vi "Get Project Members from Path - SM.vi"(6 "Shallow Scan":bool, 7 "AppRef":refnum<vi>, 8 "error in":errorcluster, 11 "Project Path":path) -> (0 "error out":errorcluster, 2 "Project Members":path[](array[path]))   [LabVIEW 2009, in "GraphicalTestRunner.lvlib"]
uses:
  GraphicalTestRunner.lvlib
  <userlib>/_OpenG.lib/array/array.llb/Remove Duplicates from 1D Array (Path)__ogtk.vi
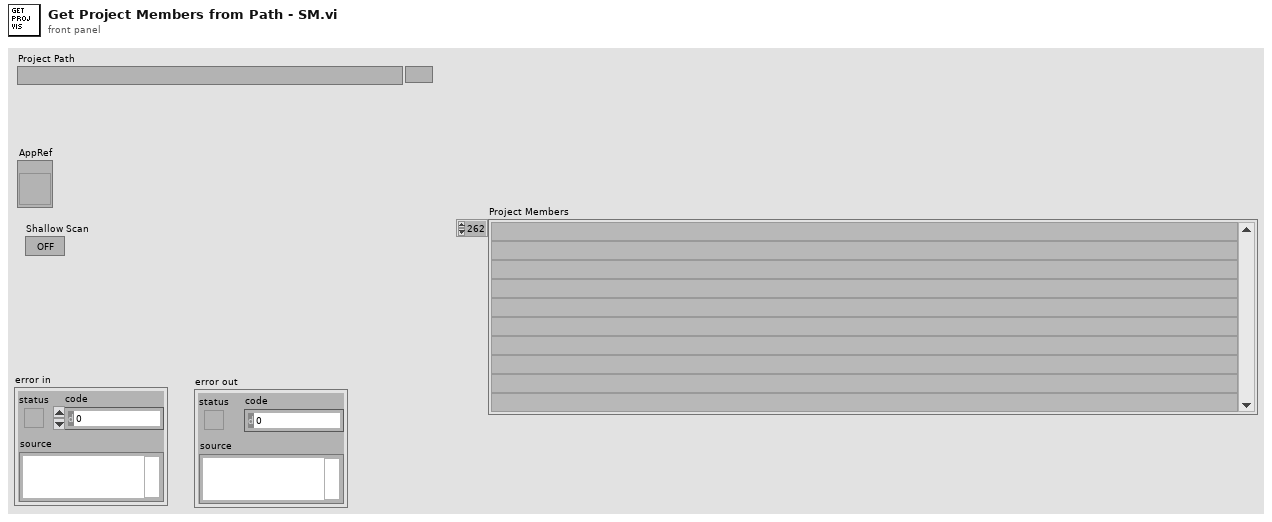
[diagram p1: front panel]
types:
  T1 = enum32{"Invalid", "Standard", "Closed", "Hidden", "Minimized", "Maximized"}
  T2 = enum32{"invalid app kind", "Development System", "Run Time System", "Student Edition", "Embedded LabVIEW", "Evaluation", "Custom"}
  T3 = cluster{"Current VI Reference":refnum<vi>, "AppRef":refnum<vi>, "Project":refnum<vi>, "My Computer":refnum<vi>, "Shallow Scan":bool, "Project Members":path[]}
  T4 = typedef "Liner Info - Cluster__jki_lib_application_control.ctl" = cluster{"path":path, "type":enum32{"Instrument", "Control", "CIN", "External subroutine", "Shared library", "Run-time menu", "Help file", "Palette menu"}, "iState":u32, "iStyle":u16, "wStyle":u16, "buttons":u16, "viflags":u32, "viflags2":u32, "links":u32[]}
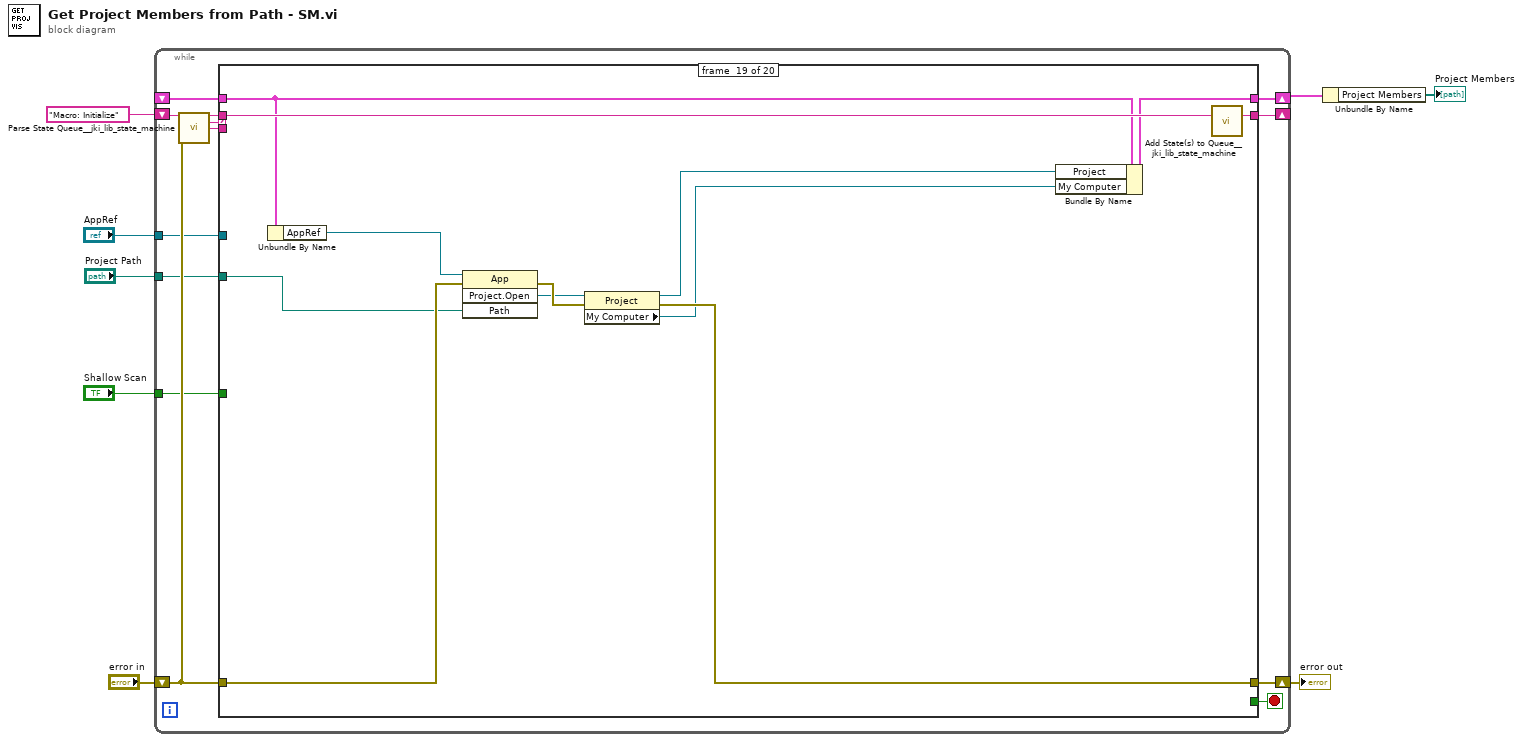
[diagram p0: block diagram]
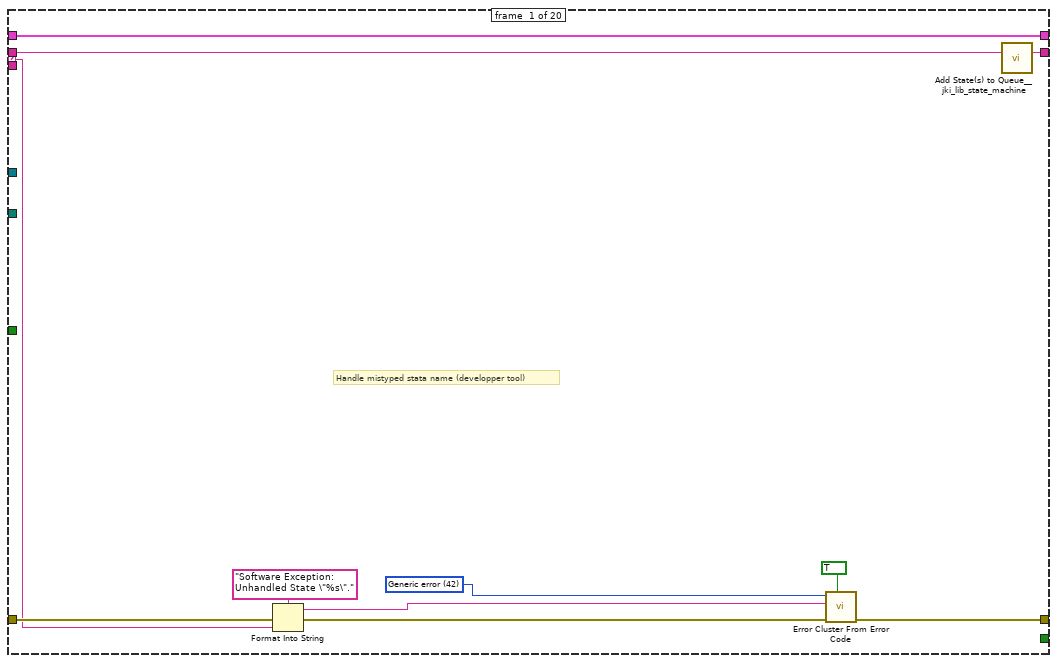
[diagram p2: hidden frame]
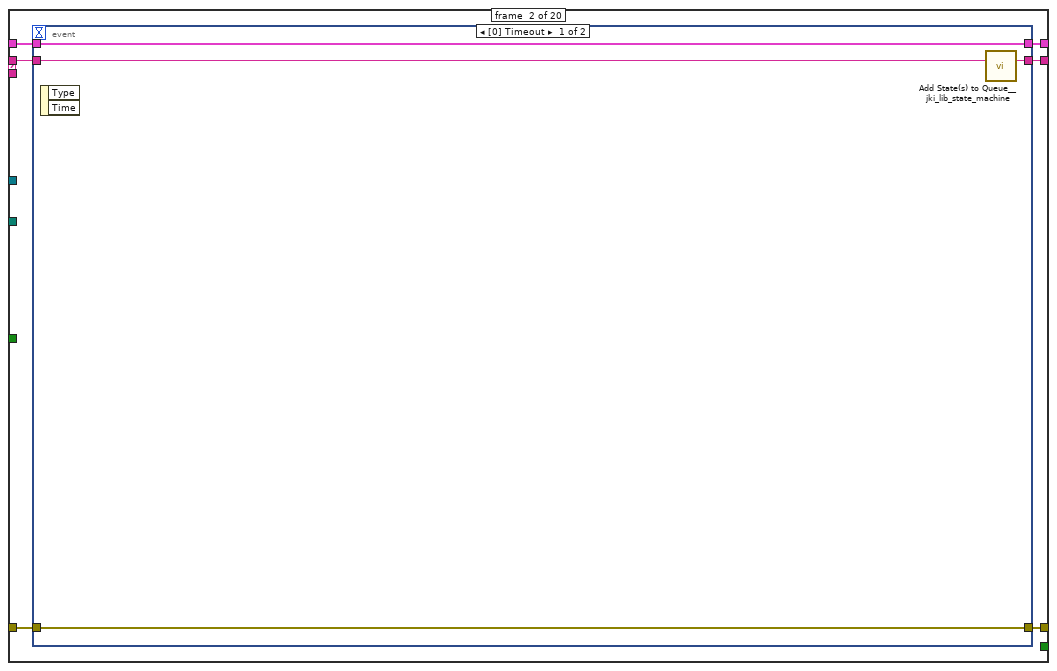
[diagram p3: hidden frame]
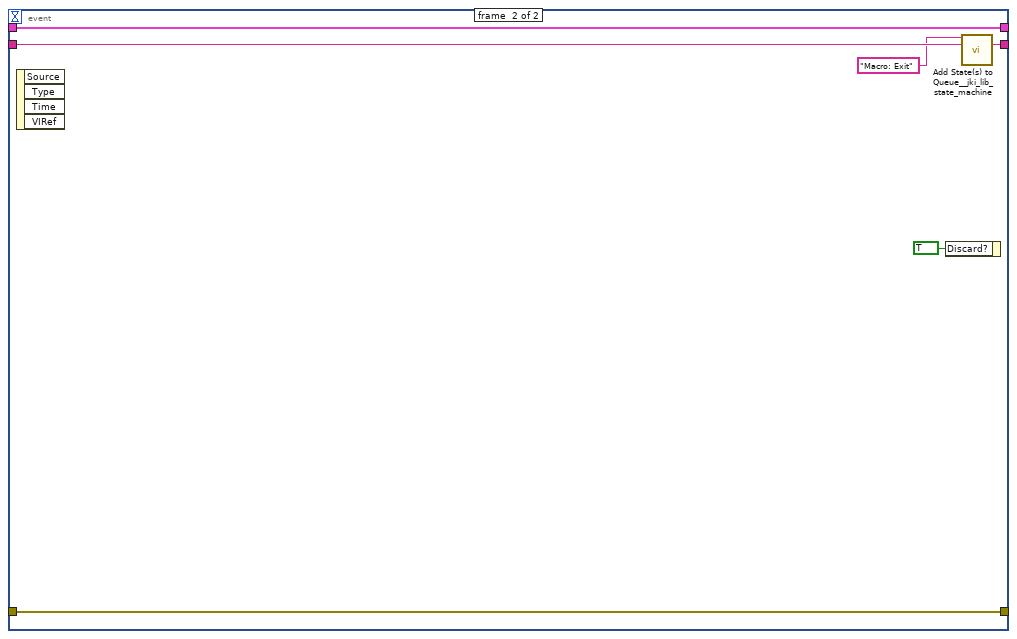
[diagram p4: hidden frame]
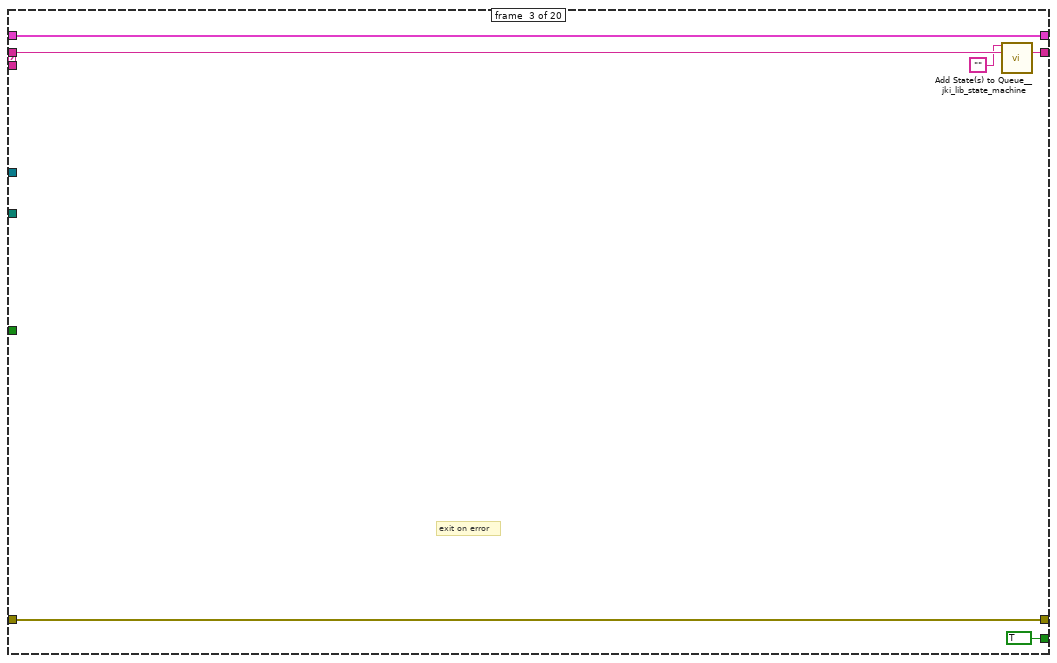
[diagram p5: hidden frame]
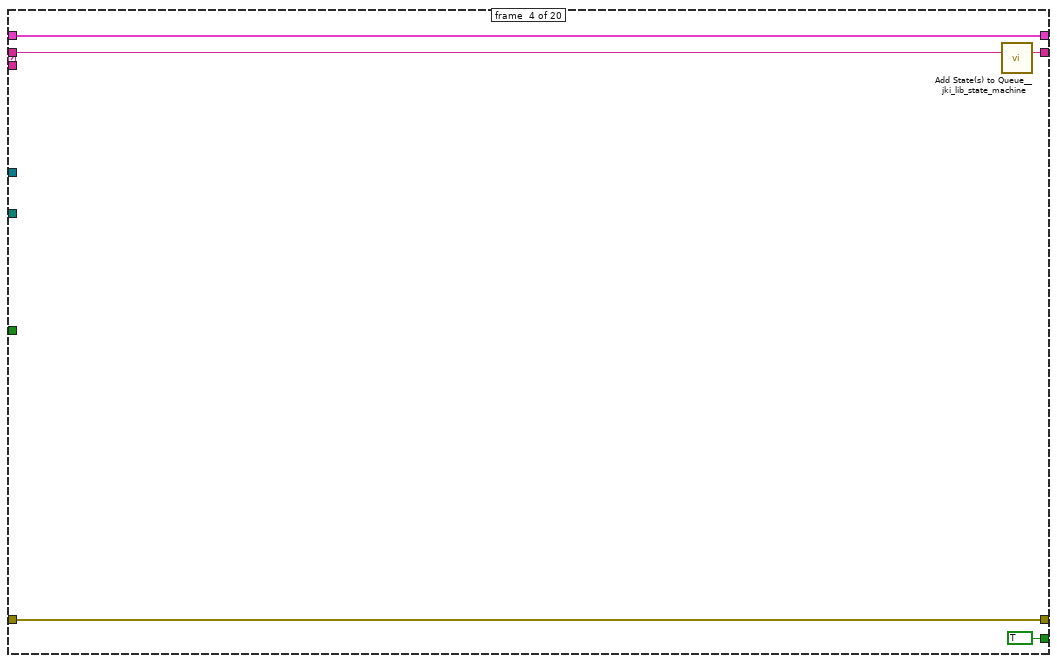
[diagram p6: hidden frame]
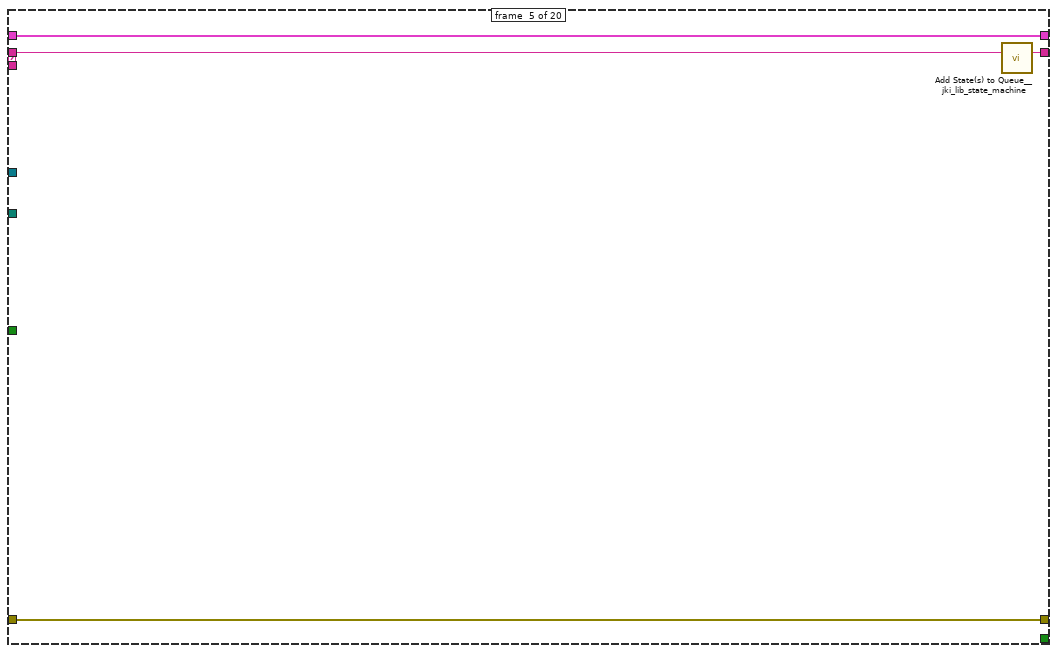
[diagram p7: hidden frame]
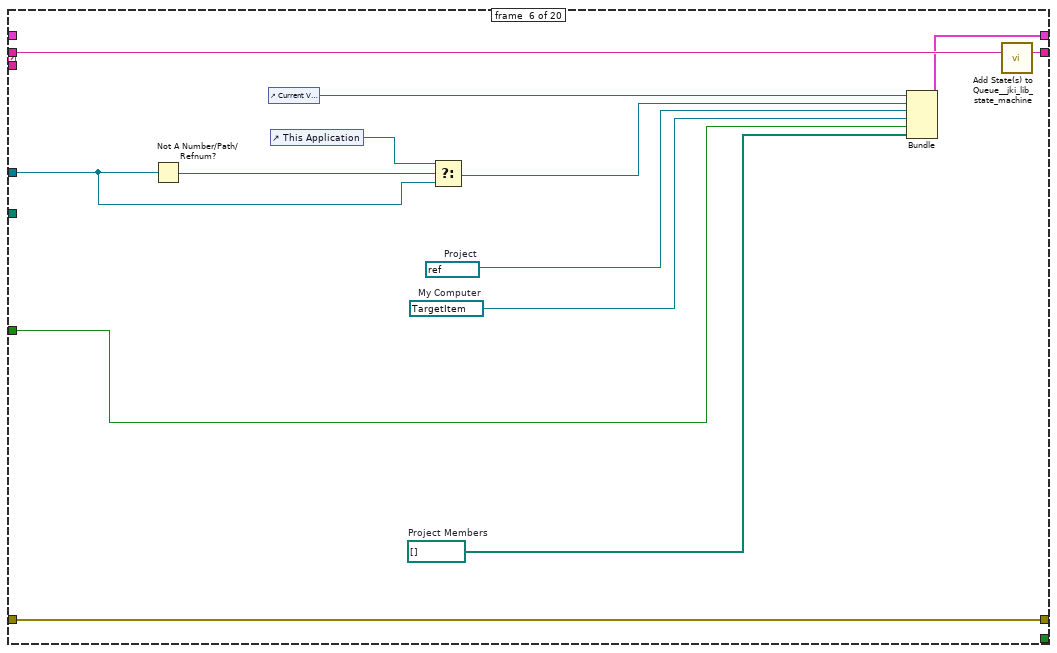
[diagram p8: hidden frame]
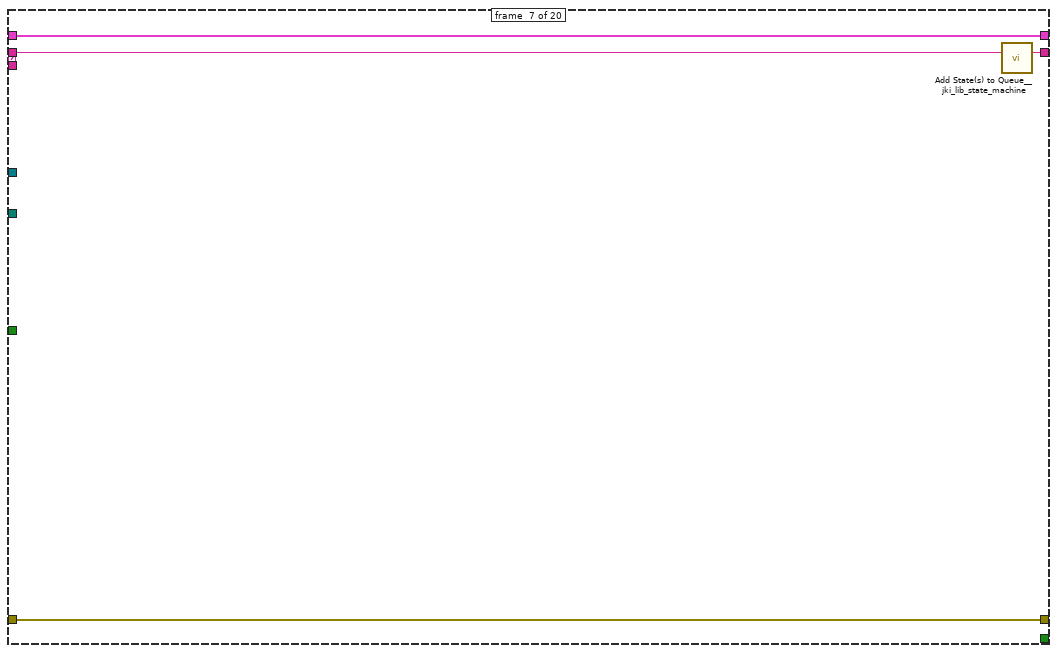
[diagram p9: hidden frame]
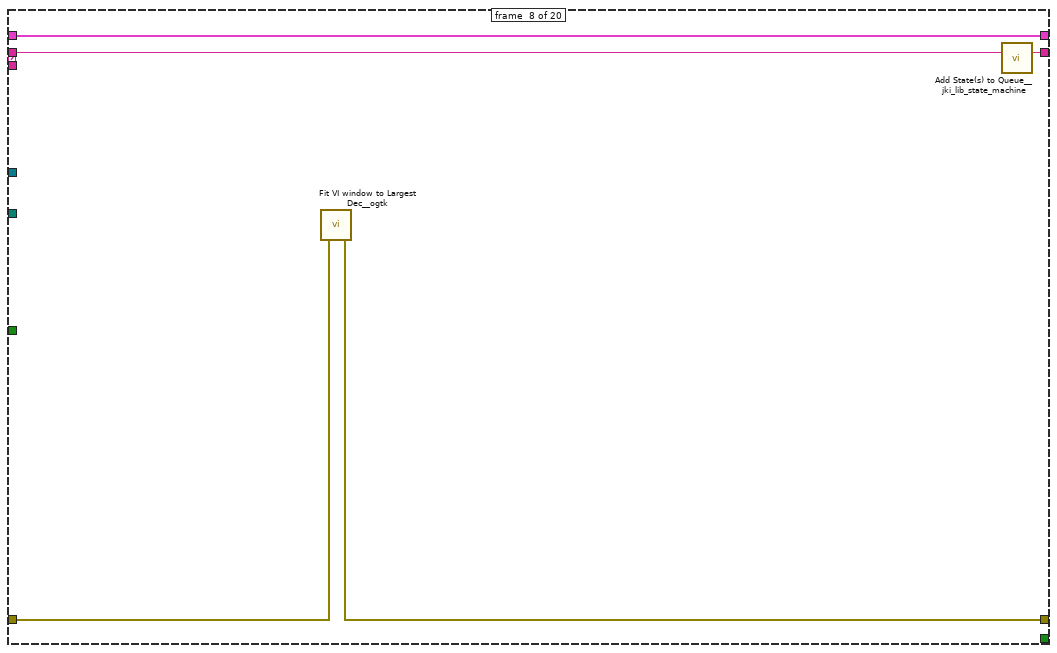
[diagram p10: hidden frame]
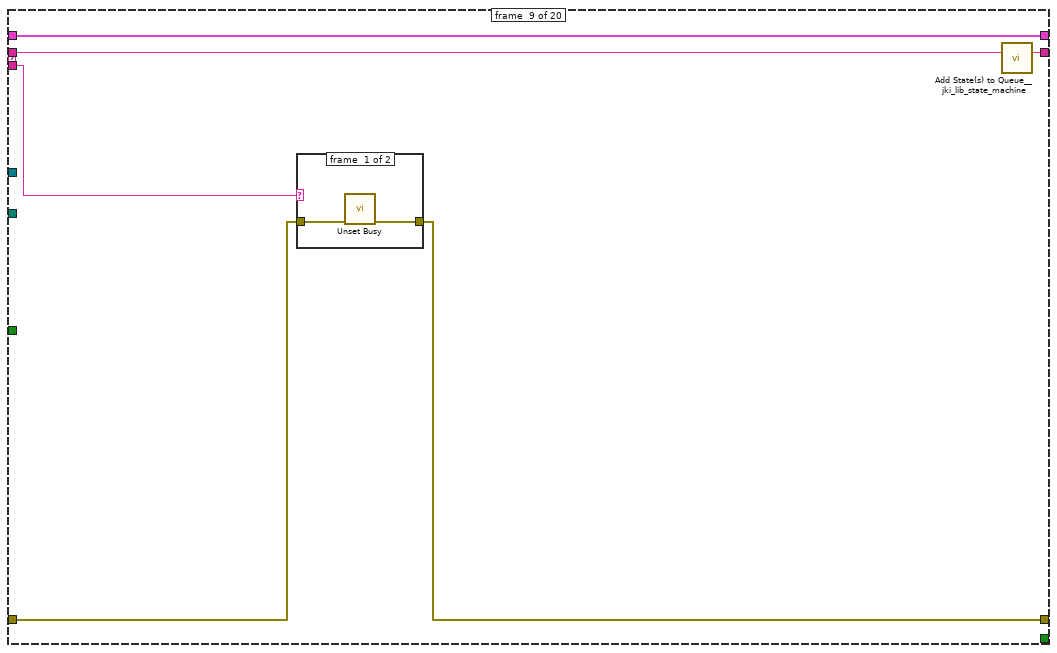
[diagram p11: hidden frame]
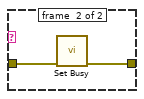
[diagram p12: hidden frame]
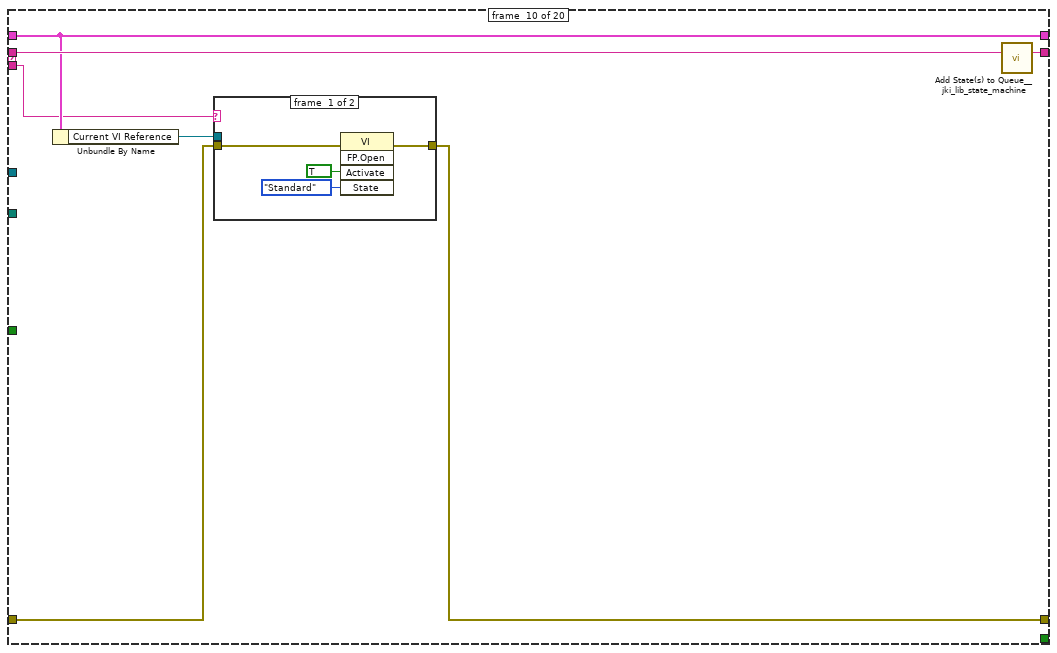
[diagram p13: hidden frame]
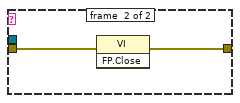
[diagram p14: hidden frame]
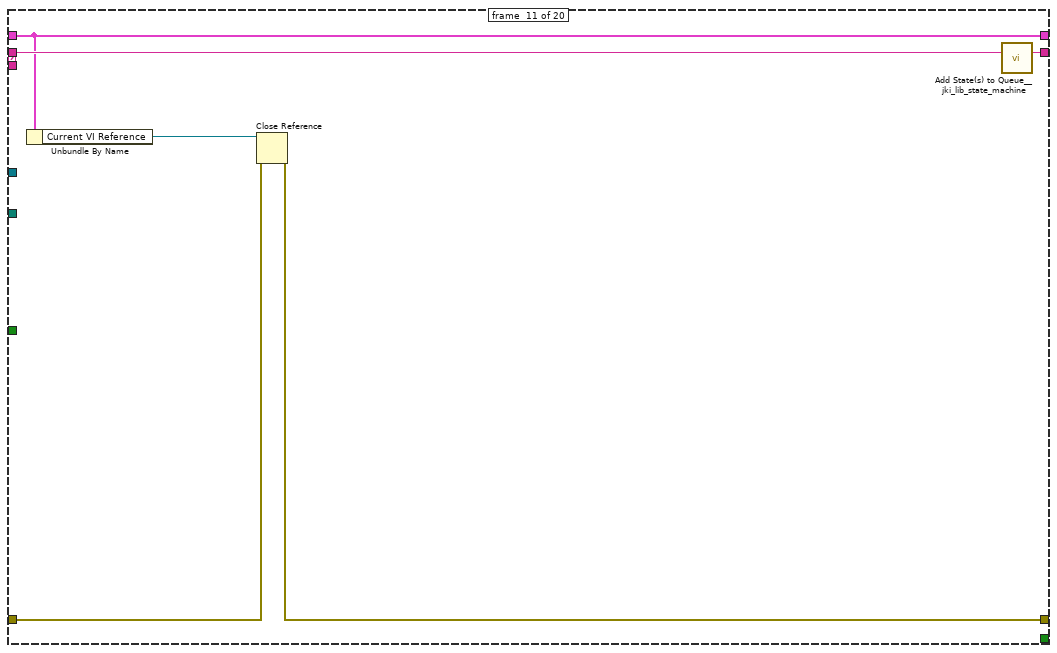
[diagram p15: hidden frame]
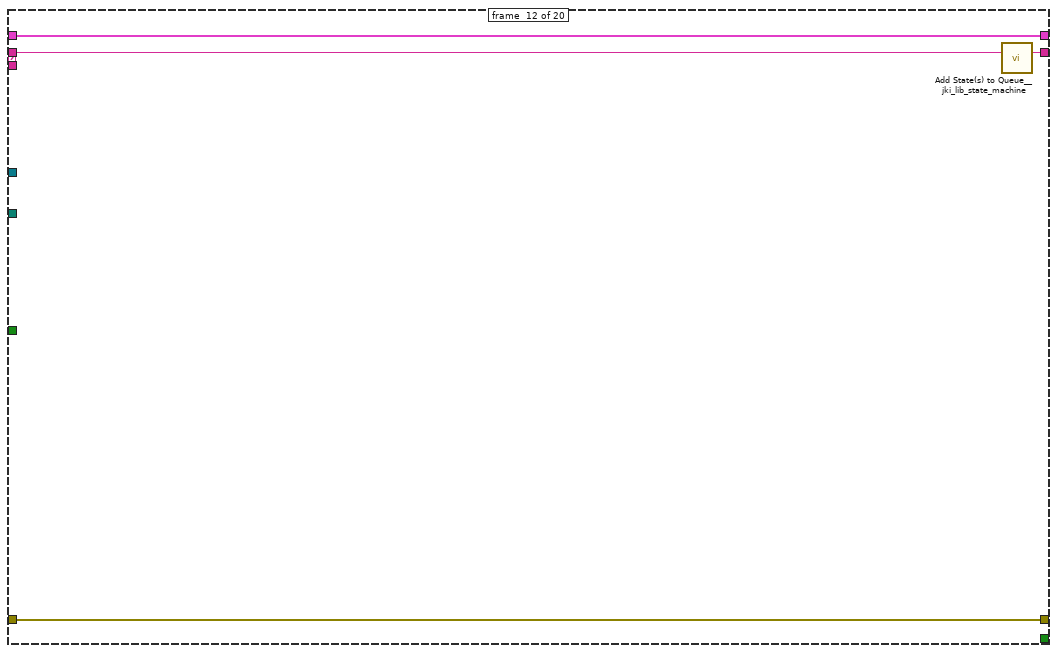
[diagram p16: hidden frame]
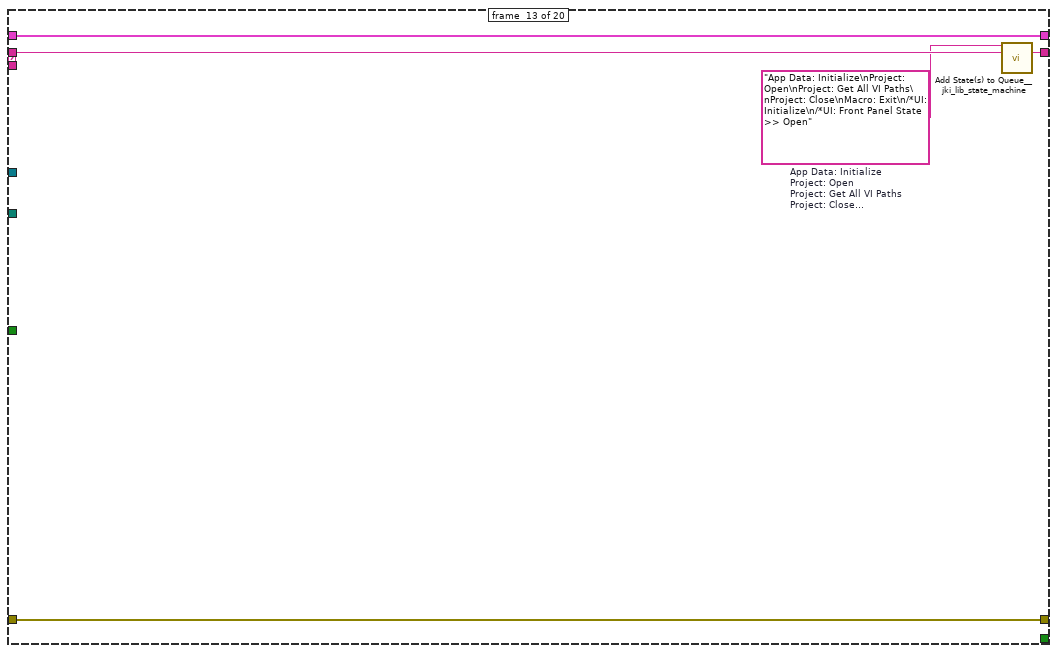
[diagram p17: hidden frame]
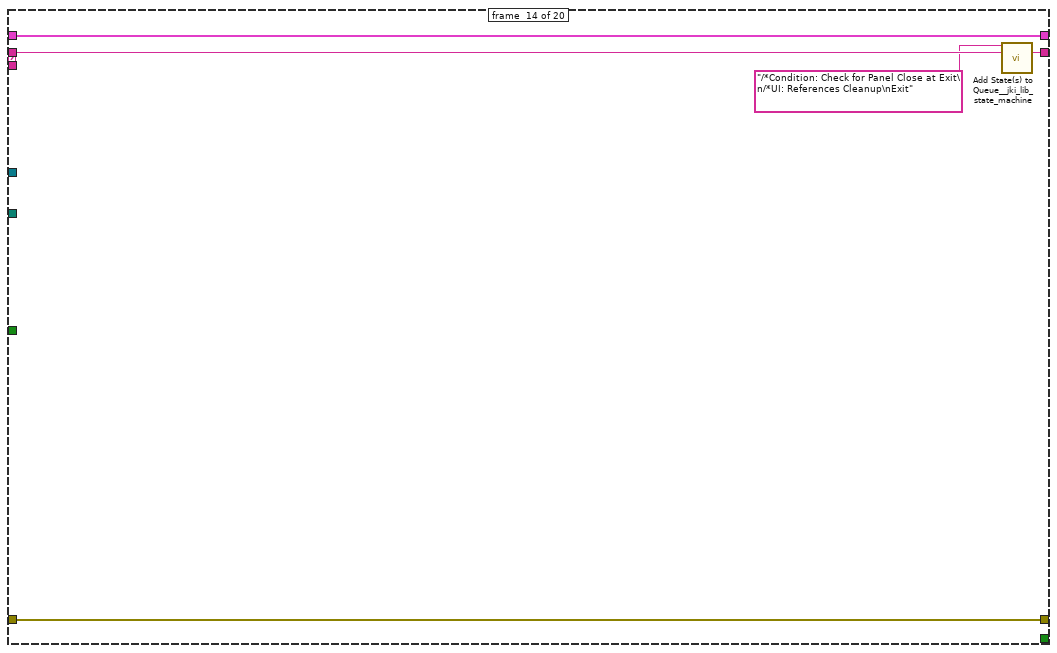
[diagram p18: hidden frame]
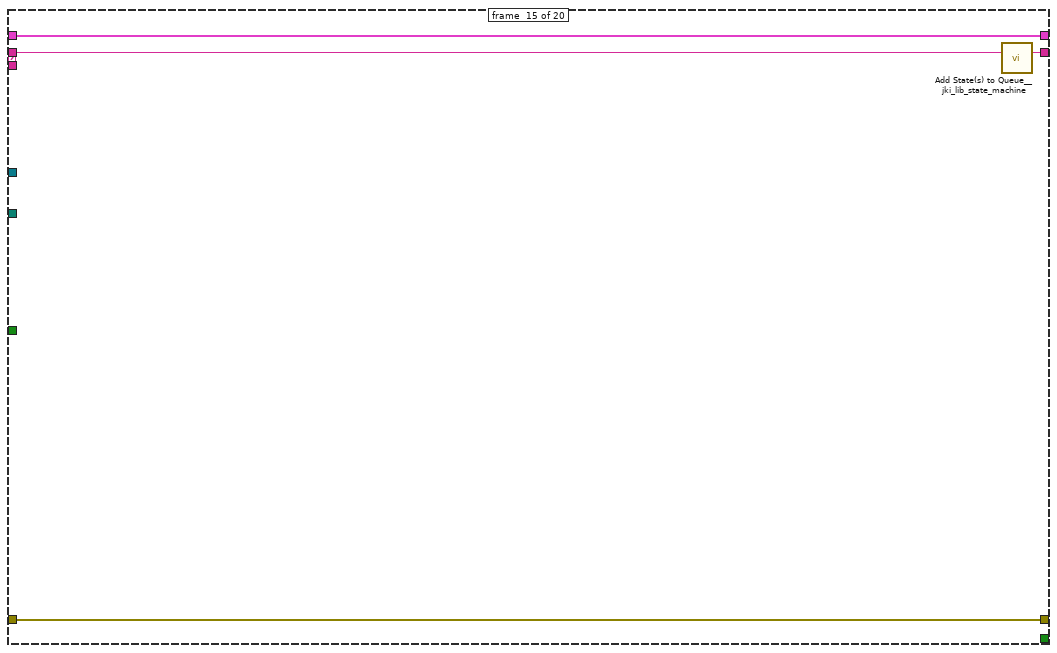
[diagram p19: hidden frame]
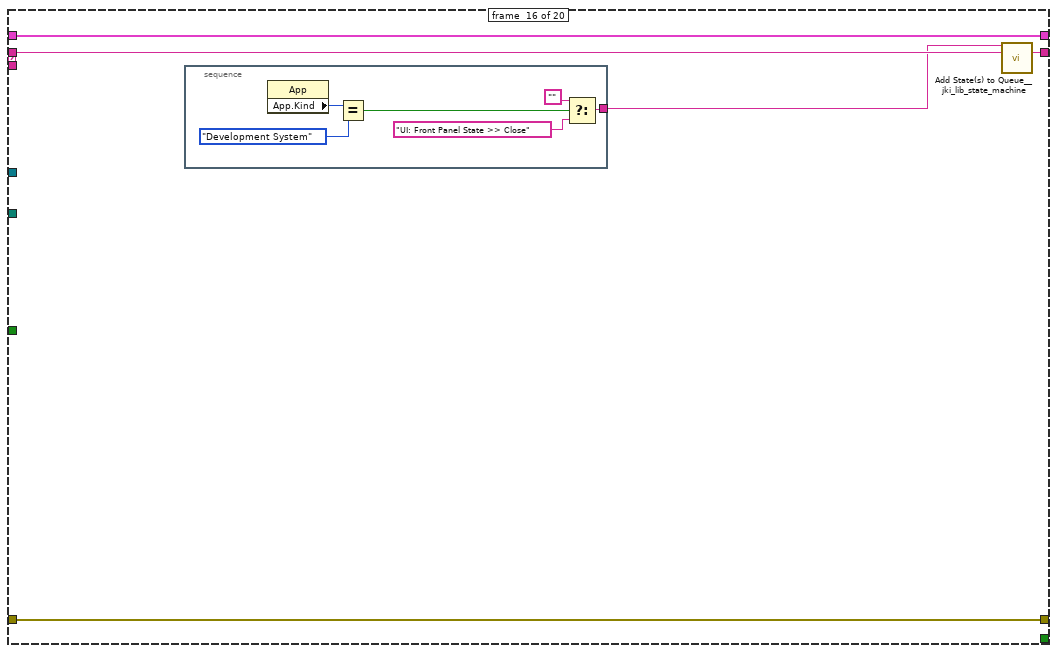
[diagram p20: hidden frame]
diagram:
  n1 = while {
    shift-right: [w12] -> w2
    shift-left: _ -> [w17]
    shift-right: [w16] -> w3
    shift-left: "error in" -> [w15]
    shift-right: [w14] -> _
    shift-left: "Macro: Initialize" -> [w18]
    tunnel: "AppRef" -> [w11]
    tunnel: "Project Path" -> [w10]
    tunnel: "Shallow Scan" -> [w9]
    stop <- w13 stop-if-true
    n2 = call <vilib>:"Parse State Queue__jki_lib_state_machine.vi"("State Queue"=w18, "Error In (no error)"=w15) -> ("Remaining States"=w20:string, "Current State"=w21:string, "Arguments"=w19:string)  [unwired: 11 in]
    n3 = case shown="\"Project: Get All VI Paths\"" w21 {
      selector: w21 -> [w26 _ _ _ _ _ _ _ _ _ _ _ _ _ _ _ _ _ _ _]
      tunnel: w20 -> [w25 w38 w54 w59 w63 w76 w80 w85 w91 w102 w114 w118 w123 w128 w132 w137 w147 w155 w167 w182]
      tunnel: w19 -> [_ _ _ _ _ _ _ _ w86 w98 _ _ _ _ _ _ _ _ _ _]
      tunnel: w17 -> [w23 w36 w51 w57 w60 _ w77 w83 w89 w99 w112 w115 w120 w125 w129 w134 w144 w153 w161 w176]
      tunnel: [w28 w35 w49 w56 w61 w74 w78 w81 w87 w96 w110 w116 w121 w126 w130 w135 w145 w150 w162 w170] -> w16
      tunnel: w15 -> [w27 w34 w49 w56 w61 w74 w78 w82 w88 w97 w111 w116 w121 w126 w130 w135 w145 w151 w163 w177]
      tunnel: [w24 w37 w53 w58 w62 w75 w79 w84 w90 w101 w113 w117 w122 w127 w131 w136 w146 w154 w166 w181] -> w14
      tunnel: [_ _ TRUE TRUE _ _ _ _ _ _ _ _ _ _ _ _ _ _ _ _] -> w13
      tunnel: [w23 w33 w51 w57 w60 w64 w77 w83 w89 w99 w112 w115 w120 w125 w129 w134 w144 w153 w160 w175] -> w12
      tunnel: w11 -> [_ _ _ _ _ w70 _ _ _ _ _ _ _ _ _ _ _ _ _ _]
      tunnel: w10 -> [_ _ _ _ _ _ _ _ _ _ _ _ _ _ _ _ _ _ w157 _]
      tunnel: w9 -> [_ _ _ _ _ w66 _ _ _ _ _ _ _ _ _ _ _ _ _ w174]
      frame #0 {
        w31 = 42 items=["No error", "Argument error", "Memory is full", "Out of zone", "End of file", "File already open", "Generic file I/O error", "File not found", "File permission error", "Disk is full", "Duplicate path", "Too many files open", "System feature not enabled", "Resource file not found", "Cannot add resource", "Resource not found", "Image not found", "Image memory error", "Pen does not exist", "Config type invalid", "Config token not found", "Config parse error", "Config memory error", "Bad external code format", "Bad external code offset", "External code not present", "Null window", "Destroy window error", "Null menu", "Print aborted", "Bad print record", "Print driver error", "Windows error during printing", "Memory error during printing", "Print dialog error", "Generic print error", "Invalid device refnum", "Device not found", "Device parameter error", "Device unit error", "Cannot open device", "Device call aborted", "Generic error", "Cancelled by user", "Object ID too low", "Object ID too high", "Object not in heap", "Unknown heap", "Unknown object (invalid DefProc)", "Unknown object (DefProc not in table)", "Message out of range", "Invalid (null) method", "Unknown message", "Manager call not supported", "Bad address", "Network operation in progress", "Network operation timed out", "Connection is busy", "Network attribute not supported", "Network error", "Address in use", "System out of memory", "Connection aborted", "Connection refused", "Not connected", "Already connected", "Connection closed", "Initialization error (interapplication manager)", "Bad occurrence", "Wait on unbound occurrence handler", "Occurrence queue overflow", "Datalog type conflict", "Unused", "Unrecognized type (interapplication manager)", "Memory corrupt", "Failed to make temporary DLL", "Old CIN version", "Drag socket not found", "Failed to load drop-object", "Failed to register OLE object", "Failed to release OLE object", "Format specifier type mismatch", "Unknown format specifier", "Too few format specifiers", "Too many format specifiers", "Scan failed", "Newer CIN version", "Error converting to variant", "Runtime menu error", "Password tampered", "Variant attribute not found", "Incompatible variant data type", "Event data is not available", "Event Store is not present", "Occurrence is not found", "Event Queue is not created", "Event info is not available", "Refnum passed is NULL", "Error retrieving Class GUID", "Error retrieving CoClass GUID", "Error retrieving TypeLib GUID.", "Bad built application magic bytes.", "Specific driver is different from the specific driver associated with the Logical Name.", "There is no session opened to the class driver.", "Max Error", "MAX - Error with config objects", "MAX - Error loading configuration", "MAX - Group not supported"]
        # "Handle mistyped stata name (developper tool)"
        n4 = Format Into String(format string="Software Exception: Unhandled State \"%s\"." ("message"), error in=w27, w26) -> (resulting string=w30:string, error out=w29:errorcluster)  [unwired: 1 in]
        n5 = call <vilib>:"Error Cluster From Error Code.vi"("show call chain? (False)"=TRUE, "error in (no error)"=w29, "error message (\"\")"=w30, "error code (0)"=w31) -> ("error out"=w28:errorcluster)  [unwired: 5 in]
        n6 = call <vilib>:"Add State(s) to Queue__jki_lib_state_machine.vi"("State(s) in (\"\")"=w25) -> ("States Out"=w24:string)  [unwired: 14 in]
      }
      frame #1 {
        n7 = event shown="[0] Timeout" {
          selector: _ -> [_ _]
          dyn-events: _ -> [_ _]
          timeout: _ -> [_ _]
          tunnel: w38 -> [w42 w48]
          tunnel: [w41 w47] -> w37
          tunnel: w36 -> [w39 w45]
          tunnel: [w40 w46] -> w35
          tunnel: w34 -> [w40 w46]
          tunnel: [w39 w45] -> w33
          event #0 {
            n8 = event-data() -> ()  [unwired: 1 in, 2 out]
            n9 = call <vilib>:"Add State(s) to Queue__jki_lib_state_machine.vi"("State(s) in (\"\")"=w42) -> ("States Out"=w41:string)  [unwired: 14 in]
          }
          event #1 {
            n10 = event-data() -> ()  [unwired: 1 in, 4 out]
            n11 = event-data("Discard?"=TRUE) -> ()  [unwired: 1 in, 1 out]
            n12 = call <vilib>:"Add State(s) to Queue__jki_lib_state_machine.vi"("State(s) in Front (\"\")"="Macro: Exit", "State(s) in (\"\")"=w48) -> ("States Out"=w47:string)  [unwired: 13 in]
          }
        }
      }
      frame #2 {
        # "exit on error"
        n13 = call <vilib>:"Add State(s) to Queue__jki_lib_state_machine.vi"("State(s) in Front (\"\")"="", "State(s) in (\"\")"=w54) -> ("States Out"=w53:string)  [unwired: 13 in]
      }
      frame #3 {
        n14 = call <vilib>:"Add State(s) to Queue__jki_lib_state_machine.vi"("State(s) in (\"\")"=w59) -> ("States Out"=w58:string)  [unwired: 14 in]
      }
      frame #4 {
        n15 = call <vilib>:"Add State(s) to Queue__jki_lib_state_machine.vi"("State(s) in (\"\")"=w63) -> ("States Out"=w62:string)  [unwired: 14 in]
      }
      frame #5 {
        w65 = path[] []  # Project Members
        w67 = refnum<vi> refnum  # My Computer
        w68 = refnum<vi> refnum  # Project
        n16 = Not A Number/Path/Refnum?(number/path/refnum=w70) -> (NaN/Path/Refnum?=w72:bool)
        n17 = control-ref of="Current VI Reference"() -> (w73:refnum<vi>)
        n18 = control-ref of="This Application"() -> (w71:refnum<vi>)
        n19 = Select(t=w71, s=w72, f=w70) -> (s? t:f=w69:refnum<vi>)
        n20 = Bundle("Current VI Reference"=w73, "AppRef"=w69, "Project"=w68, "My Computer"=w67, "Shallow Scan"=w66, "Project Members"=w65) -> (w64:T3)  [unwired: 1 in]
        n21 = call <vilib>:"Add State(s) to Queue__jki_lib_state_machine.vi"("State(s) in (\"\")"=w76) -> ("States Out"=w75:string)  [unwired: 14 in]
      }
      frame #6 {
        n22 = call <vilib>:"Add State(s) to Queue__jki_lib_state_machine.vi"("State(s) in (\"\")"=w80) -> ("States Out"=w79:string)  [unwired: 14 in]
      }
      frame #7 {
        n23 = call <userlib>:"Fit VI window to Largest Dec__ogtk.vi"("error in (no error)"=w82) -> ("error out"=w81:errorcluster)  [unwired: 5 in, 1 out]
        n24 = call <vilib>:"Add State(s) to Queue__jki_lib_state_machine.vi"("State(s) in (\"\")"=w85) -> ("States Out"=w84:string)  [unwired: 14 in]
      }
      frame #8 {
        n25 = case shown="\"Idle\", Default" w86 {
          tunnel: w88 -> [w93 w95]
          tunnel: [w92 w94] -> w87
          frame #0 {
            n26 = call <vilib>:"Unset Busy.vi"("error in (no error)"=w93) -> ("error out"=w92:errorcluster)  [unwired: 10 in]
          }
          frame #1 {
            n27 = call <vilib>:"Set Busy.vi"("error in (no error)"=w95) -> ("error out"=w94:errorcluster)  [unwired: 9 in, 1 out]
          }
        }
        n28 = call <vilib>:"Add State(s) to Queue__jki_lib_state_machine.vi"("State(s) in (\"\")"=w91) -> ("States Out"=w90:string)  [unwired: 14 in]
      }
      frame #9 {
        n29 = Unbundle By Name(w99) -> ("Current VI Reference"=w100:refnum<vi>)
        n30 = case shown="\"Close\"" w98 {
          tunnel: w100 -> [_ _]
          tunnel: w97 -> [w104 w108]
          tunnel: [w103 w107] -> w96
          frame #0 {
            n31 = invoke class="VI" method="FP.Open"(error in=w104, "Activate"=TRUE, "State"=T1."Standard") -> (error out=w103:errorcluster)  [unwired: 2 in, 4 out]
          }
          frame #1 {
            n32 = invoke class="VI" method="FP.Close"(error in=w108) -> (error out=w107:errorcluster)  [unwired: 2 in, 2 out]
          }
        }
        n33 = call <vilib>:"Add State(s) to Queue__jki_lib_state_machine.vi"("State(s) in (\"\")"=w102) -> ("States Out"=w101:string)  [unwired: 14 in]
      }
      frame #10 {
        n34 = Unbundle By Name(w112) -> ("Current VI Reference"=w109:refnum<vi>)
        n35 = Close Reference(reference=w109, error in (no error)=w111) -> (error out=w110:errorcluster)
        n36 = call <vilib>:"Add State(s) to Queue__jki_lib_state_machine.vi"("State(s) in (\"\")"=w114) -> ("States Out"=w113:string)  [unwired: 14 in]
      }
      frame #11 {
        n37 = call <vilib>:"Add State(s) to Queue__jki_lib_state_machine.vi"("State(s) in (\"\")"=w118) -> ("States Out"=w117:string)  [unwired: 14 in]
      }
      frame #12 {
        w119 = "App Data: Initialize\nProject: Open\nProject: Get All VI Paths\nProject: Close\nMacro: Exit\n/*UI: Initialize\n/*UI: Front Panel State >> Open"  # App Data: Initialize Project: Open Project: Get All VI Paths Project: Close Macro: Exit /*UI: Initialize /*UI: Front Panel State >> Open
        n38 = call <vilib>:"Add State(s) to Queue__jki_lib_state_machine.vi"("State(s) in Front (\"\")"=w119, "State(s) in (\"\")"=w123) -> ("States Out"=w122:string)  [unwired: 13 in]
      }
      frame #13 {
        n39 = call <vilib>:"Add State(s) to Queue__jki_lib_state_machine.vi"("State(s) in Front (\"\")"="/*Condition: Check for Panel Close at Exit\n/*UI: References Cleanup\nExit", "State(s) in (\"\")"=w128) -> ("States Out"=w127:string)  [unwired: 13 in]
      }
      frame #14 {
        n40 = call <vilib>:"Add State(s) to Queue__jki_lib_state_machine.vi"("State(s) in (\"\")"=w132) -> ("States Out"=w131:string)  [unwired: 14 in]
      }
      frame #15 {
        n41 = stacked-sequence {
          tunnel: [w143] -> w133
          frame #0 {
            n42 = property class="App"() -> ("App.Kind"=w140:T2)  [unwired: 2 in, 2 out]
            n43 = Equal?(x=w140, y=T2."Development System") -> (x = y?=w139:bool)
            n44 = Select(t="", s=w139, f="UI: Front Panel State >> Close") -> (s? t:f=w143:string)
          }
        }
        n45 = call <vilib>:"Add State(s) to Queue__jki_lib_state_machine.vi"("State(s) in Front (\"\")"=w133, "State(s) in (\"\")"=w137) -> ("States Out"=w136:string)  [unwired: 13 in]
      }
      frame #16 {
        n46 = call <vilib>:"Add State(s) to Queue__jki_lib_state_machine.vi"("State(s) in (\"\")"=w147) -> ("States Out"=w146:string)  [unwired: 14 in]
      }
      frame #17 {
        n47 = Unbundle By Name(w153) -> ("Project"=w148:refnum<vi>, "My Computer"=w149:refnum<vi>)
        n48 = Close Reference(reference=w149, error in (no error)=w151) -> (error out=w152:errorcluster)
        n49 = Close Reference(reference=w148, error in (no error)=w152) -> (error out=w150:errorcluster)
        n50 = call <vilib>:"Add State(s) to Queue__jki_lib_state_machine.vi"("State(s) in (\"\")"=w155) -> ("States Out"=w154:string)  [unwired: 14 in]
      }
      frame #18 {
        n51 = Unbundle By Name(w161) -> ("AppRef"=w156:refnum<vi>)
        n52 = invoke class="App" method="Project.Open"(reference=w156, error in=w163, "Path"=w157) -> (error out=w165:errorcluster, "Project:Open"=w164:refnum<vi>)  [unwired: 1 in, 2 out]
        n53 = property class="Project"(reference=w164, error in=w165) -> (reference out=w159:refnum<vi>, error out=w162:errorcluster, "My Computer"=w158:refnum<vi>)
        n54 = Bundle By Name(cluster=w161, "Project"=w159, "My Computer"=w158) -> (w160:T3)
        n55 = call <vilib>:"Add State(s) to Queue__jki_lib_state_machine.vi"("State(s) in (\"\")"=w167) -> ("States Out"=w166:string)  [unwired: 14 in]
      }
      frame #19 {
        n56 = Unbundle By Name(w176) -> ("AppRef"=w172:refnum<vi>, "My Computer"=w169:refnum<vi>)
        n57 = invoke class="TargetItem" method="Get All Descendents"(reference=w169, error in=w177, "Type"="VI") -> (error out=w178:errorcluster, "All Descendents"=w179:refnum<vi>[])  [unwired: 4 in, 5 out]
        n58 = for {
          tunnel: w179 -> [w198] mode=indexing
          shift-right: [w196] -> w171
          shift-left: w178 -> [w197]
          tunnel: [w194] -> w168 mode=indexing
          n59 = property class="ProjectItem"(reference=w198, error in=w197) -> (reference out=w195:refnum<vi>, error out=w196:errorcluster, "Path"=w194:path)
          n60 = Close Reference(reference=w195) -> ()  [unwired: 1 in, 1 out]
        }
        n61 = case "shallow scan?" shown="False" w174 {
          tunnel: w168 -> [w189 w193]
          tunnel: [w186 w193] -> w173
          tunnel: w172 -> [w183 _]
          tunnel: w171 -> [w185 w192]
          tunnel: [w184 w192] -> w170
          frame #0 {
            n62 = call <vilib>:"Read VI Hierarchy on Disk__jki_lib_application_control.vi"("error in"=w185, "Paths to Read"=w189, "application reference (local)"=w183) -> ("error out"=w184:errorcluster, "Linker Info"=w188:T4[])  [unwired: 5 in, 2 out]
            n63 = for {
              tunnel: w188 -> [w191] mode=indexing
              tunnel: [w190] -> w187 mode=indexing
              n64 = Unbundle By Name(w191) -> ("path"=w190:path)
            }
            n65 = call-poly <userlib>:"Remove Duplicates from 1D Array__ogtk.vi"("Input Array"=w187) -> ("Output Array"=w186:path[])  [unwired: 1 out]
          }
          frame #1 {
          }
        }
        n66 = Bundle By Name(cluster=w176, "Project Members"=w173) -> (w175:T3)
        n67 = call <vilib>:"Add State(s) to Queue__jki_lib_state_machine.vi"("State(s) in (\"\")"=w182) -> ("States Out"=w181:string)  [unwired: 14 in]
      }
    }
  }
  "error out" <- w3
  n68 = Unbundle By Name(w2) -> ("Project Members"=→"Project Members":path[])
